vi "rt_loop_system_health_monitoring.vi"(11 "Message Queue":refnum<queue> caption="消息队列") -> ()   [LabVIEW 2015]
uses:
  support_vis/message_queue/message_cluster.ctl
  globals/global_all_rt_loop_stop.vi
  globals/global_configuration_options.vi
  globals/global_rt_stream_connections.vi
  <vilib>/nisyscfg/Close (System).vi
  <vilib>/nisyscfg/nisyscfg.lvlib
  <resource>/objmgr/nisysapi.rc
  <vilib>/NI_Real-Time Target Support.lvlib
  support_vis/message_queue/message_queue.lvlib
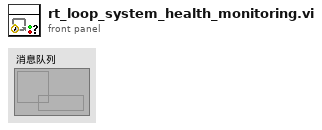
[diagram p1: front panel]
types:
  T1 = typedef "NI_Real-Time Target Support.lvlib/RT CPU Load.ctl" = cluster{"Total (%)":dbl, "Time Critical (%)":dbl, "Timed Structures (%)":dbl, "High (%)":dbl, "Above Normal (%)":dbl, "Normal (%)":dbl, "Background (%)":dbl, "Idle (%)":dbl, "ISR (%)":dbl}
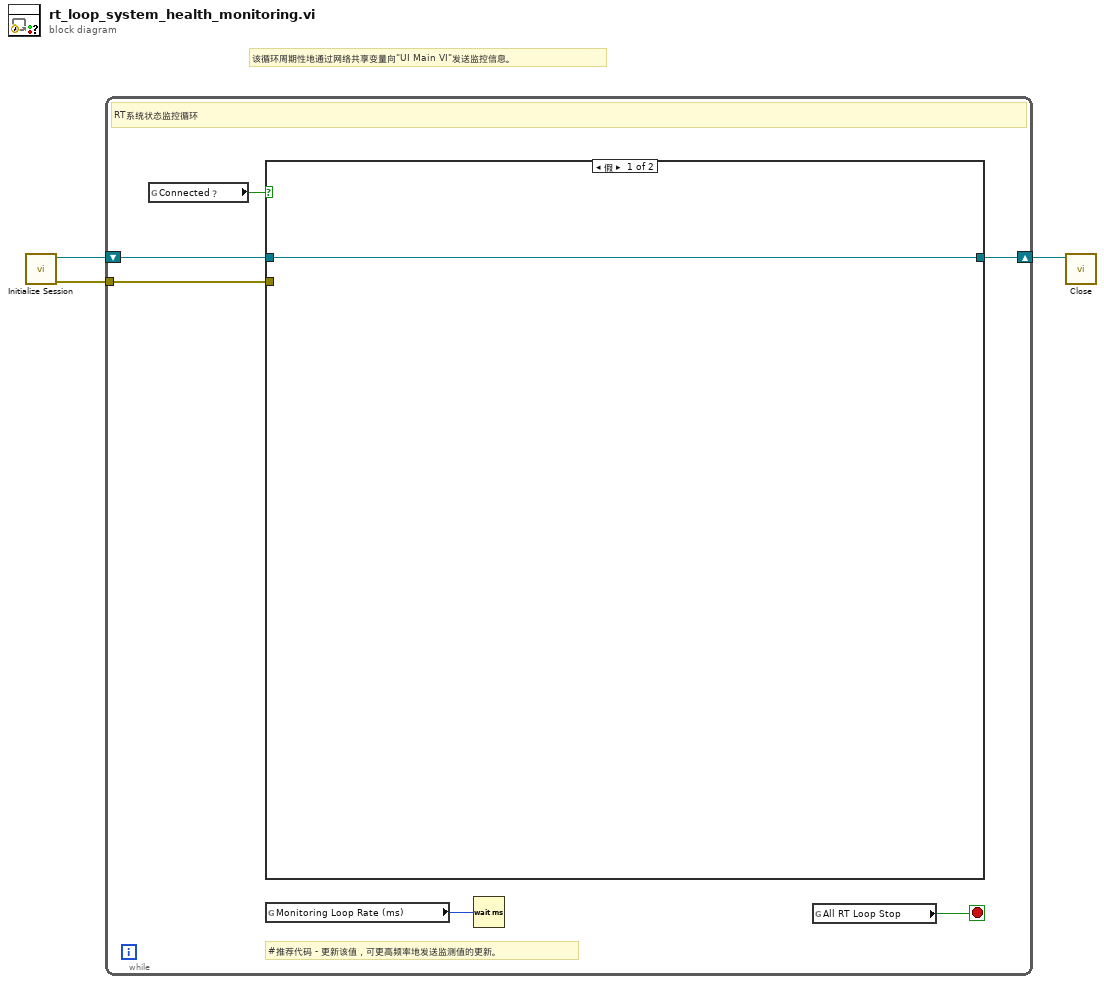
[diagram p0: block diagram]
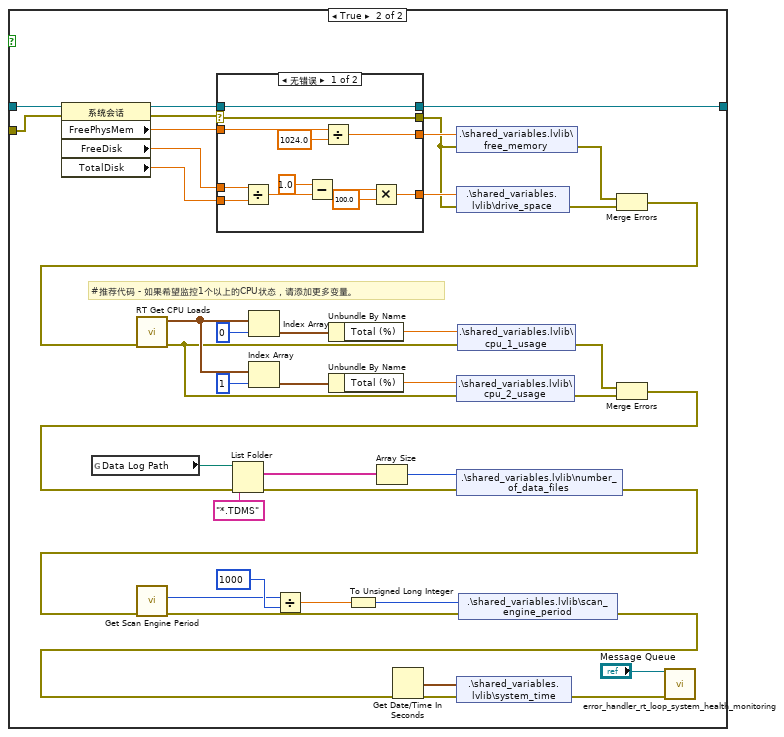
[diagram p2: hidden frame]
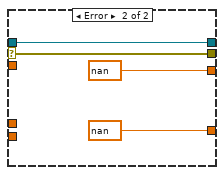
[diagram p3: hidden frame]
diagram:
  # "该循环周期性地通过网络共享变量向\"UI Main VI\"发送监控信息。"
  n1 = call <vilib>:"Initialize Session.vi"() -> ("error out"=w1:errorcluster, "Session out"=w3:refnum<k21>)  [unwired: 10 in]
  n2 = while {
    shift-right: [w7] -> w2
    shift-left: w3 -> [w8]
    tunnel: w1 -> [w5]
    stop <- w9 stop-if-true
    # "#推荐代码 - 更新该值，可更高频率地发送监测值的更新。"
    # "RT系统状态监控循环"
    n3 = global read "global_rt_stream_connections.vi" "Connected？"() -> (w4:bool)
    n4 = case shown="假" w4 {
      tunnel: w8 -> [w10 w31]
      tunnel: [w10 w42] -> w7
      tunnel: w5 -> [_ w30]
      frame False {
      }
      frame True {
        # "#推荐代码 - 如果希望监控1个以上的CPU状态，请添加更多变量。"
        n5 = property class="系统会话"(reference=w31, error in=w30) -> (reference out=w27:refnum<k21>, error out=w26:errorcluster, "FreePhysMem"=w25:dbl, "FreeDisk"=w24:dbl, "TotalDisk"=w23:dbl)
        n6 = global read "global_configuration_options.vi" "Data Log Path"() -> (w48:path)
        n7 = case shown="无错误" w26 {
          selector: w26 -> [w61 w65]
          tunnel: w25 -> [w60 _]
          tunnel: [w62 nan] -> w29
          tunnel: [w61 w65] -> w17
          tunnel: w24 -> [w59 _]
          tunnel: w23 -> [w58 _]
          tunnel: [w57 nan] -> w28
          tunnel: w27 -> [w51 w63]
          tunnel: [w51 w63] -> w42
          frame No Error {
            # "将千字节转换为字节"
            n8 = Divide(x=w59, y=w58) -> (x/y=w53:dbl)
            n9 = Subtract(x=1.0, y=w53) -> (x-y=w52:dbl)
            n10 = Divide(x=w60, y=1024.0 ("x")) -> (x/y=w62:dbl)
            n11 = Multiply(x=w52, y=100.0 ("x")) -> (x*y=w57:dbl)
          }
          frame Error {
            # "不支持的属性。"
          }
        }
        n12 = Get Date/Time In Seconds() -> (seconds since 1Jan1904=w41:timestamp)
        n13 = shared-variable ".\\shared_variables.lvlib\\free_memory"(w29, error in=w17) -> (error out=w15:errorcluster)
        n14 = shared-variable ".\\shared_variables.lvlib\\drive_space"(w28, error in=w17) -> (error out=w16:errorcluster)
        n15 = Merge Errors(w15, w16) -> (w14:errorcluster)
        n16 = call <vilib>:"RT Get CPU Loads.vi"("error in (no error)"=w14) -> ("error out"=w19:errorcluster, "CPU loads"=w20:T1[])  [unwired: 9 in]
        n17 = Index Array(array=w20, index=0 ("索引")) -> (element=w50:T1)
        n18 = Index Array(array=w20, index=1 ("索引")) -> (element=w22:T1)
        n19 = Unbundle By Name(w50) -> ("Total (%)"=w49:dbl)
        n20 = Unbundle By Name(w22) -> ("Total (%)"=w18:dbl)
        n21 = shared-variable ".\\shared_variables.lvlib\\cpu_2_usage"(w18, error in=w19) -> (error out=w13:errorcluster)
        n22 = shared-variable ".\\shared_variables.lvlib\\cpu_1_usage"(w49, error in=w19) -> (error out=w12:errorcluster)
        n23 = Merge Errors(w12, w13) -> (w11:errorcluster)
        n24 = List Folder(path=w48, pattern="*.TDMS", error in=w11) -> (filenames=w45:string[], error out=w47:errorcluster)  [unwired: 1 in, 2 out]
        n25 = Array Size(array=w45) -> (size(s)=w46:i32)
        n26 = shared-variable ".\\shared_variables.lvlib\\number_of_data_files"(w46, error in=w47) -> (error out=w33:errorcluster)
        n27 = call <vilib>:"Get Scan Engine Period.vi"("error in (no error)"=w33) -> ("scan period (uSec)"=w35:u32, "error out"=w34:errorcluster)  [unwired: 13 in]
        n28 = Divide(x=w35, y=u32 1000) -> (x/y=w37:dbl)
        n29 = To Unsigned Long Integer(number=w37) -> (unsigned 32bit integer=w38:u32)
        n30 = shared-variable ".\\shared_variables.lvlib\\scan_engine_period"(w38, error in=w34) -> (error out=w32:errorcluster)
        n31 = shared-variable ".\\shared_variables.lvlib\\system_time"(w41, error in=w32) -> (error out=w39:errorcluster)
        n32 = call "error_handler_rt_loop_system_health_monitoring.vi"("error in (no error)"=w39, "Message Queue"="Message Queue") -> ()  [unwired: 9 in, 1 out]
      }
    }
    n33 = global read "global_configuration_options.vi" "Monitoring Loop Rate (ms)"() -> (w6:u32)
    n34 = Wait (ms)(milliseconds to wait=w6) -> ()  [unwired: 1 out]
    n35 = global read "global_all_rt_loop_stop.vi" "All RT Loop Stop"() -> (w9:bool)
  }
  n36 = call-poly <vilib>:"Close.vi"("Session in"=w2) -> ()  [unwired: 10 in, 1 out]
